vi "Read LCR Meter.lvclass.vi"(11 "LCR-Measurement in":refnum<class "LCR-Meas.lvclass">) -> (2 "LCR Meter.lvclass":refnum<class "LCR Meter.lvclass">, 3 "LCR-Measurement out":refnum<class "LCR-Meas.lvclass">)   [LabVIEW 2020, in "LCR-Meas.lvclass"]
uses:
  LCR-Meas.lvclass
  Instruments/LCR Meter/LCR Meter.lvclass
  LCR-Meas.lvclass/LCR-Meas.ctl
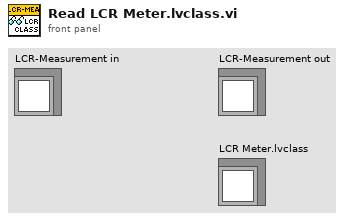
[diagram p1: front panel]
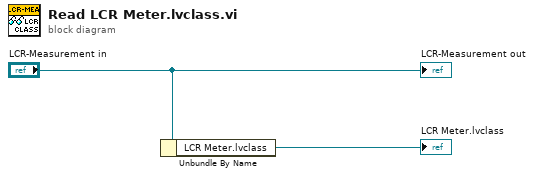
[diagram p0: block diagram]
diagram:
  n1 = Unbundle By Name("LCR-Measurement in") -> ("LCR Meter.lvclass"=→"LCR Meter.lvclass":refnum<class "LCR Meter.lvclass">)
  "LCR-Measurement out" <- "LCR-Measurement in"
